vi "tsapp_get_bus_statistics_AllInfo.vi"(8 "错误输入（无错误）":errorcluster, 10 "AIdxChn":T2(ring), 11 "ABusType":enum16{"APP_CAN", "APP_LIN"}(ring)) -> (0 "错误输出":errorcluster, 3 "TLIBCANBusStatistics_Ctrl":T1)   [LabVIEW 2016]
uses:
  TLIBCANBusStatistics_Ctrl.ctl
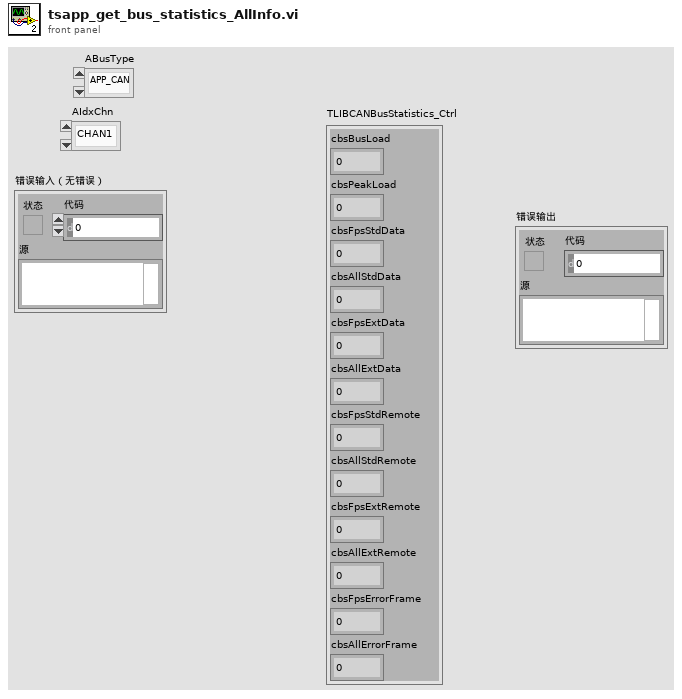
[diagram p1: front panel]
types:
  T1 = typedef "TLIBCANBusStatistics_Ctrl.ctl" = cluster{"cbsBusLoad":dbl, "cbsPeakLoad":dbl, "cbsFpsStdData":dbl, "cbsAllStdData":dbl, "cbsFpsExtData":dbl, "cbsAllExtData":dbl, "cbsFpsStdRemote":dbl, "cbsAllStdRemote":dbl, "cbsFpsExtRemote":dbl, "cbsAllExtRemote":dbl, "cbsFpsErrorFrame":dbl, "cbsAllErrorFrame":dbl}
  T2 = enum16{"CHAN1", "CHAN2", "CHAN3", "CHAN4", "CHAN5", "CHAN6", "CHAN7", "CHAN8", "CHAN9", "CHAN10", "CHAN11", "CHAN12", "CHAN13", "CHAN14", "CHAN15", "CHAN16"}
  T3 = enum16{"cbsBusLoad", "cbsPeakLoad", "cbsFpsStdData", "cbsAllStdData", "cbsFpsExtData", "cbsAllExtData", "cbsFpsStdRemote", "cbsAllStdRemote", "cbsFpsExtRemote", "cbsAllExtRemote", "cbsFpsErrorFrame", "cbsAllErrorFrame"}
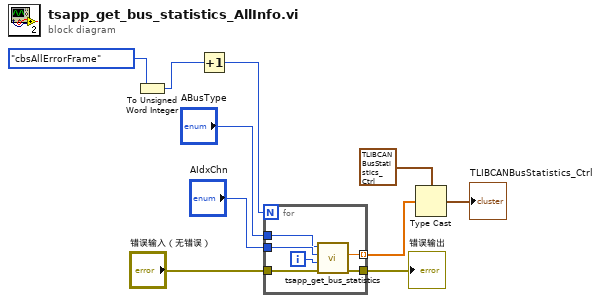
[diagram p0: block diagram]
diagram:
  n1 = To Unsigned Word Integer(number=T3."cbsAllErrorFrame" ("TLIBCANBusStatistics")) -> (unsigned 16bit integer=w1:u16)
  n2 = Increment(x=w1) -> (x+1=w10:u16)
  n3 = for {
    N: w10 -> [_]
    tunnel: "AIdxChn" -> [w15]
    tunnel: "ABusType" -> [w14]
    tunnel: [w13] -> w7 mode=indexing
    tunnel: [w12] -> w3
    tunnel: "错误输入（无错误）" -> [w11]
    i -> [w16]
    n4 = call "tsapp_get_bus_statistics.vi"("错误输入（无错误）"=w11, "TLIBCANBusStatistics"=w16, "AIdxChn"=w15, "ABusType"=w14) -> ("错误输出"=w12:errorcluster, "AStat"=w13:dbl)  [unwired: 5 in, 1 out]
  }
  "错误输出" <- w3
  n5 = Type Cast(type=T1 {"cbsBusLoad"=0.0, "cbsPeakLoad"=0.0, "cbsFpsStdData"=0.0, "cbsAllStdData"=0.0, "cbsFpsExtData"=0.0, "cbsAllExtData"=0.0, "cbsFpsStdRemote"=0.0, "cbsAllStdRemote"=0.0, "cbsFpsExtRemote"=0.0, "cbsAllExtRemote"=0.0, "cbsFpsErrorFrame"=0.0, "cbsAllErrorFrame"=0.0} ("TLIBCANBusStatistics_Ctrl"), x=w7) -> (*(type *) &x=→"TLIBCANBusStatistics_Ctrl":T1)
